vi "Close.vi"(8 "error in (no error)":errorcluster, 11 "Carya Config (Buffer) in":refnum<class "CConfig Nonpersistant Buffer.lvclass">) -> (0 "error out":errorcluster)   [LabVIEW 2013, in "CConfig Nonpersistant Buffer.lvclass"]
doc: "Copyright 2018, Carya Automatisering, Wiebe Walstra."
uses:
  CConfig Nonpersistant Buffer.lvclass
  CConfig Nonpersistant Buffer.lvclass/CConfig Nonpersistant Buffer.ctl
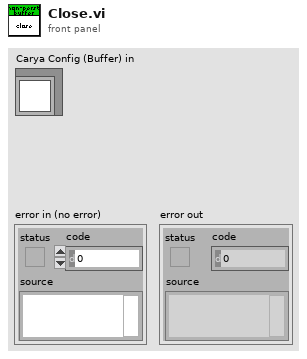
[diagram p1: front panel]
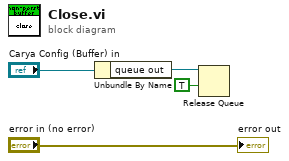
[diagram p0: block diagram]
diagram:
  n1 = Unbundle By Name("Carya Config (Buffer) in") -> ("queue out"=w2:refnum<queue>)
  n2 = Release Queue(queue=w2, force destroy? (F)=TRUE) -> ()  [unwired: 1 in, 3 out]
  "error out" <- "error in (no error)"
